vi "OpenProjectTxtWithCode.vi"   [LabVIEW 2020]
doc: "Allow to open the project.txt with VS Code to edit the order of the Tools menu."
uses:
  846b9cc9-b277-4677-9e2a-d5b282abfd94.vi
  <resource>/dialog/lvconfig.llb/LV Config Read String.vi
types:
  T1 = enum32{"Invalid", "Standard", "Closed", "Hidden", "Minimized", "Maximized"}
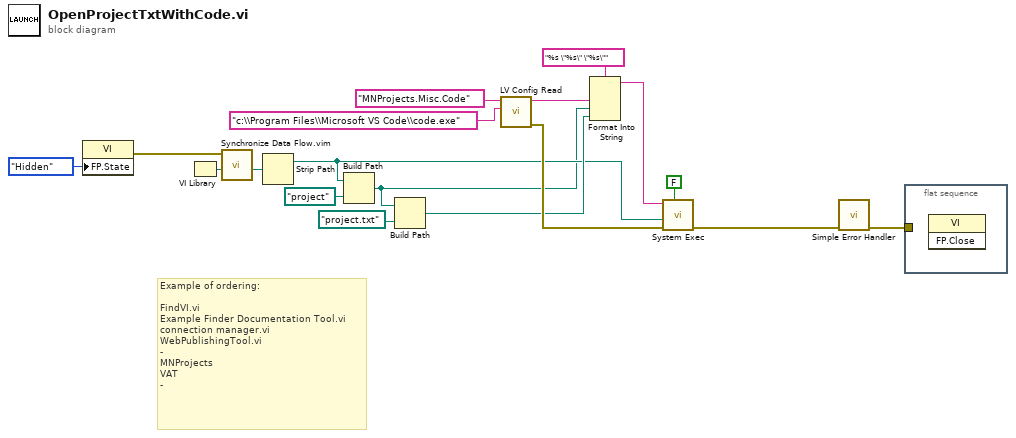
[diagram p0: block diagram]
diagram:
  # "Example of ordering:\n\nFindVI.vi\nExample Finder Documentation Tool.vi\nconnection manager.vi\nWebPublishingTool.vi\n-\nMNProjects\nVAT\n-"
  n1 = property class="VI"("FP.State"=T1."Hidden" ("Front Panel Window:State")) -> (error out=w5:errorcluster)  [unwired: 2 in, 1 out]
  n2 = VI Library() -> (path=w9:path)
  n3 = call "Synchronize Data Flow.vim"("input 3"=w9, "input 1"=w5) -> ("output 3"=w7:path)  [unwired: 2 in, 3 out]
  n4 = Strip Path(path=w7) -> (stripped path=w3:path)  [unwired: 1 out]
  n5 = Build Path(base path=w3, name or relative path=path "project") -> (appended path=w1:path)
  n6 = Build Path(base path=w1, name or relative path=path "project.txt") -> (appended path=w4:path)
  n7 = call-poly <resource>:"LV Config Read.vi"("default value"="c:\\Program Files\\Microsoft VS Code\\code.exe" ("command line"), "key"="MNProjects.Misc.Code") -> ("error out"=w14:errorcluster, "value"=w11:string)  [unwired: 3 in, 1 out]
  n8 = Format Into String(format string="%s \"%s\" \"%s\"", w11, w1, w4) -> (resulting string=w10:string)  [unwired: 2 in, 1 out]
  n9 = call <vilib>:"System Exec.vi"("wait until completion? (T)"=FALSE, "error in (no error)"=w14, "working directory"=w3, "command line"=w10) -> ("error out"=w17:errorcluster)  [unwired: 4 in, 3 out]
  n10 = call <vilib>:"Simple Error Handler.vi"("error in (no error)"=w17) -> ("error out"=w13:errorcluster)  [unwired: 4 in, 4 out]
  n11 = flat-sequence {
    tunnel: w13 -> [_]
    frame #0 {
      n12 = invoke class="VI" method="FP.Close"() -> ()  [unwired: 3 in, 3 out]
    }
  }
